vi "Door Open.vi"(8 "stop":bool, 11 "Enum":enum16{"Unlock Door", "Lock Door"}(ring)) -> (3 "Status":bool)   [LabVIEW 2014]
panel:
  # "OPEN DOOR TO CONTINUE"
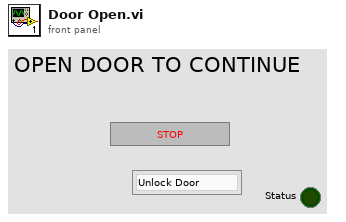
[diagram p1: front panel]
types:
  T1 = enum16{"P6.0", "P6.1", "P6.2", "P6.3", "P6.4", "P6.5", "P6.6", "P6.7", "P7.0", "P7.1", "P7.2", "P7.3", "P7.4", "P7.5", "P7.6", "P7.7", "P8.0", "P8.1", "P8.2", "P8.3", "P8.4", "P8.5", "P8.6", "P8.7", "P9.0", "P9.1", "P9.2", "P9.3", "P9.4", "P9.5", "P9.6", "P9.7", "11.0", "11.1", "11.2", "11.3", "11.4", "11.5", "11.6", "11.7", "Init"}
  T2 = enum16{"Init Pneumatic Relays", "Pneumatic_Drive_0", "Pneumatic_Drive_1", "Pneumatic_Drive_2", "Pneumatic_Drive_3", "Pneumatic_Drive_4", "Pneumatic_Drive_5", "Pneumatic_Drive_6", "Pneumatic_Drive_7", "Pneumatic_Drive_8", "Pneumatic_Drive_9", "Pneumatic_Drive_10", "Pneumatic_Drive_11", "Pneumatic_Drive_12", "Pneumatic_Drive_13", "Pneumatic_Drive_14", "Pneumatic_Drive_15"}
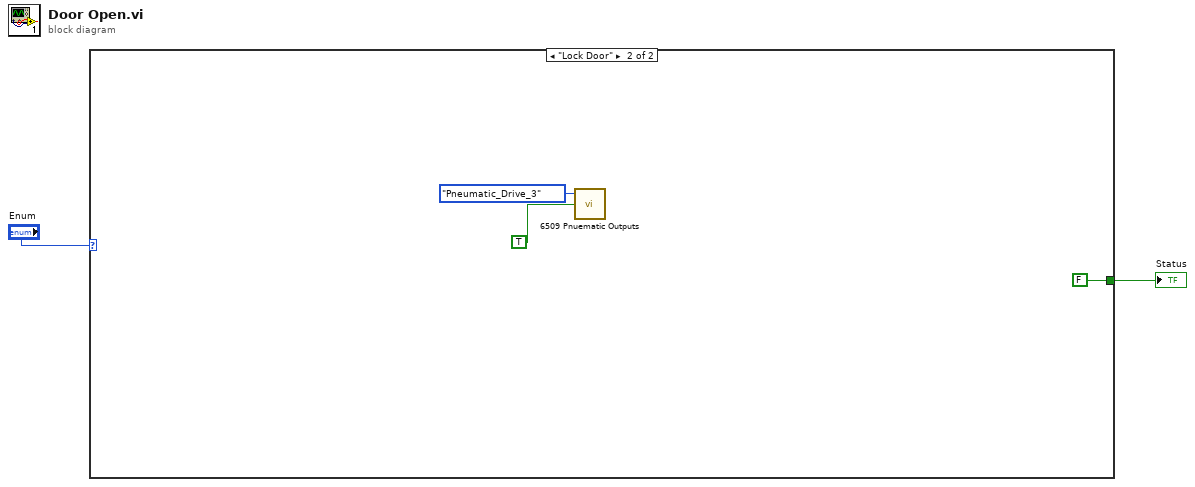
[diagram p0: block diagram]
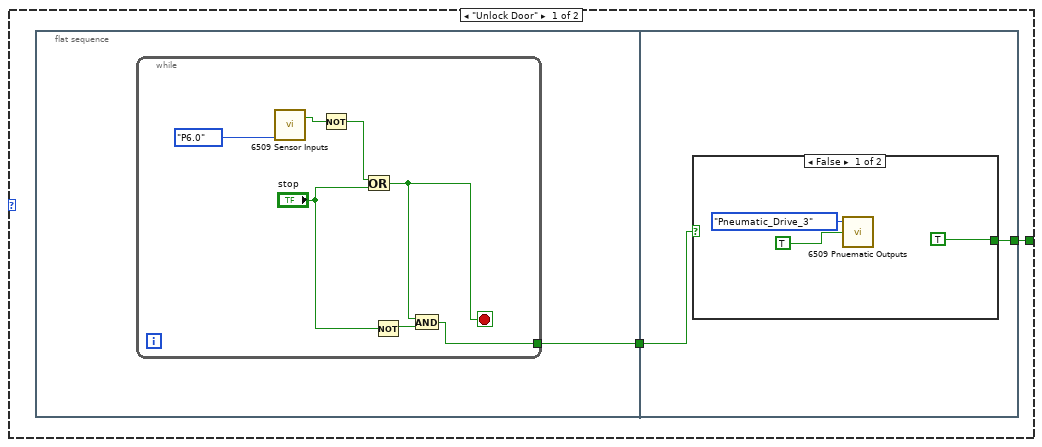
[diagram p2: hidden frame]
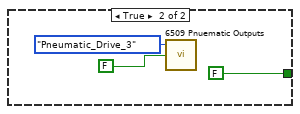
[diagram p3: hidden frame]
diagram:
  n1 = case shown="\"Lock Door\"" "Enum" {
    tunnel: [w3 FALSE ("Status")] -> w1
    frame "Unlock Door" {
      n2 = flat-sequence {
        tunnel: [w5] -> w4
        tunnel: w4 -> [w14]
        tunnel: [w13] -> w3
        frame #0 {
          n3 = while {
            tunnel: [w8] -> w5
            stop <- w6 stop-if-true
            n4 = call "6509 Sensor Inputs.vi"("Enum"=T1."P6.0" ("Enum 2")) -> ("State"=w12:bool)  [unwired: 1 in, 1 out]
            n5 = Not(x=w12) -> (.not. x?=w11:bool)
            n6 = Or(x=w11, y="stop") -> (x .or. y?=w6:bool)
            n7 = Not(x="stop") -> (.not. x?=w9:bool)
            n8 = And(x=w6, y=w9) -> (x .and. y?=w8:bool)
          }
        }
        frame #1 {
          n9 = case shown="False" w14 {
            tunnel: [TRUE ("Status") FALSE ("Status")] -> w13
            frame False {
              n10 = call "6509 Pnuematic Outputs.vi"("Enable Output"=TRUE ("Enable Relays"), "Enum"=T2."Pneumatic_Drive_3") -> ()  [unwired: 1 in, 1 out]
            }
            frame True {
              n11 = call "6509 Pnuematic Outputs.vi"("Enable Output"=FALSE ("Enable Relays"), "Enum"=T2."Pneumatic_Drive_3") -> ()  [unwired: 1 in, 1 out]
            }
          }
        }
      }
    }
    frame "Lock Door" {
      n12 = call "6509 Pnuematic Outputs.vi"("Enable Output"=TRUE ("Enable Relays"), "Enum"=T2."Pneumatic_Drive_3") -> ()  [unwired: 1 in, 1 out]
    }
  }
  "Status" <- w1
